vi "Split 1D Array.vi"(5 "JSON Value in":refnum<class "JSON Value.lvclass">, 9 "index":i32, 11 "error in (no error)":errorcluster) -> (6 "JSON Value out":refnum<class "JSON Value.lvclass">, 10 "JSON Value out":refnum<class "JSON Value.lvclass">, 15 "error out":errorcluster)   [LabVIEW 2016, in "JSON Value.lvclass"]
doc: "Divides array at index and returns the two portions with the element of index at the beginning of second subarray."
uses:
  JSON Value.lvclass
  JSON Value.lvclass/JSON Value.ctl
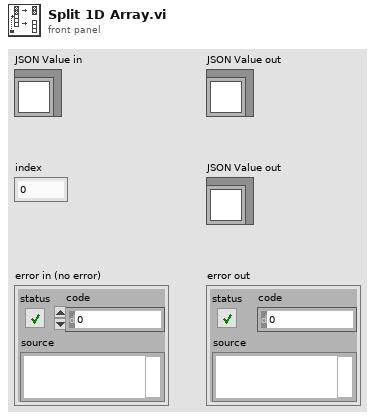
[diagram p1: front panel]
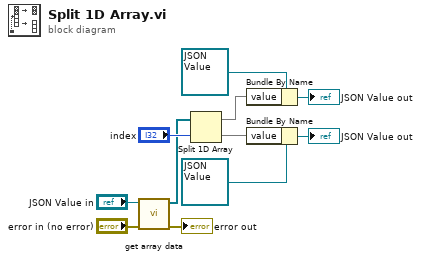
[diagram p0: block diagram]
diagram:
  n1 = call "get array data.vi"("error in (no error)"="error in (no error)", "JSON Value in"="JSON Value in") -> ("error out"=→"error out":errorcluster, "JSON Array out"=w4:refnum<class "JSON Value.lvclass">[])  [unwired: 8 in]
  n2 = Split 1D Array(array=w4, index="index") -> (first subarray=w8:refnum<class "JSON Value.lvclass">[], second subarray=w7:refnum<class "JSON Value.lvclass">[])
  n3 = Bundle By Name(cluster=refnum<class "JSON Value.lvclass"> refnum ("JSON Object in"), "value"=w8) -> (→"JSON Value out":refnum<class "JSON Value.lvclass">)
  n4 = Bundle By Name(cluster=refnum<class "JSON Value.lvclass"> refnum ("JSON Object in"), "value"=w7) -> (→"JSON Value out":refnum<class "JSON Value.lvclass">)
